vi "Cannon Stow.vi"(1 "Cannon Info In":T2) -> (0 "Cannon Info Out":T2)   [LabVIEW 2013]
uses:
  <vilib>/Rock Robotics/WPI/Relay/WPI_RelayValue.ctl
  <vilib>/Rock Robotics/WPI/Solenoid/WPI_SolenoidValue.ctl
  Intake/Intake Global.vi
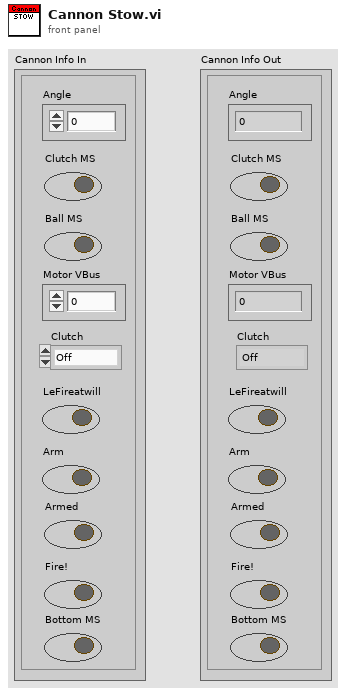
[diagram p1: front panel]
types:
  T1 = typedef "WPI_RelayValue.ctl" = enum16{"Off", "On", "Forward", "Reverse"}
  T2 = cluster{"Angle":dbl, "Clutch MS":bool, "Ball MS":bool, "Motor VBus":dbl, "Clutch ":T1, "LeFireatwill":bool, "Arm":bool, "Armed":bool, "Fire!":bool, "Bottom MS":bool}
  T3 = typedef "WPI_SolenoidValue.ctl" = enum16{"Off", "On", "Forward", "Reverse"}
  T4 = cluster{"Arm State":bool, "Gripper Out":bool, "Gripper Execution":T1, "Arm Execution":T3, "Gripper In":bool}
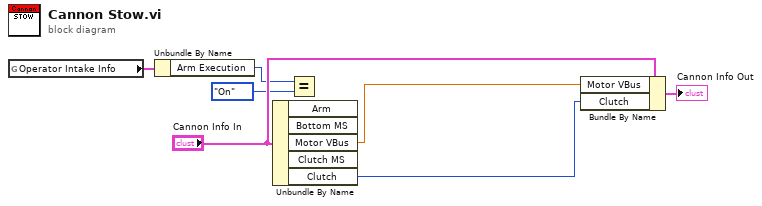
[diagram p0: block diagram]
diagram:
  n1 = global read "Intake Global.vi" "Operator Intake Info"() -> (w5:T4)
  n2 = Unbundle By Name(w5) -> ("Arm Execution"=w3:T3)
  n3 = Unbundle By Name("Cannon Info In") -> ("Motor VBus"=w2:dbl, "Clutch"=w1:T1)  [unwired: 3 out]
  n4 = Equal?(x=w3, y=WPI_SolenoidValue."On" ("Arm Execution")) -> ()  [unwired: 1 out]
  n5 = Bundle By Name(cluster="Cannon Info In", "Motor VBus"=w2, "Clutch"=w1) -> (→"Cannon Info Out":T2)
